vi "MC5e Calculate_Squad.vi"(6 "index":i32, 7 "Mode":T1, 11 "Input Squad":T3={"Squad Name"="", "# Soldiers"=1, "Battle Rating"=0, "Flying"=FALSE, "Mounted"=FALSE, "Speed"=3, "Range"=1, "Morale"=0, "Max Endurance"=10, "Current Endurance"=10, "Size"=enum."Medium", "Space Taken"=1, "Difficult Terrain"=[0, 1, 3, 6, 7], "CR"=1, "Special / Notes"=""} {"CR" items=["30", "29", "28", "27", "26", "25", "24", "23", "22", "21", "20", "19", "18", "17", "16", "15", "14", "13", "12", "11", "10", "9", "8", "7", "6", "5", "4", "3", "2", "1", "1/2", "1/4", "1/8"]}) -> (2 "OK Button Disabled?":T2(ring), 3 "output squad":T3={"Squad Name"="", "# Soldiers"=1, "Battle Rating"=0, "Flying"=FALSE, "Mounted"=FALSE, "Speed"=3, "Range"=1, "Morale"=0, "Max Endurance"=10, "Current Endurance"=10, "Size"=enum."Medium", "Space Taken"=1, "Difficult Terrain"=[0, 1, 3, 6, 7], "CR"=1, "Special / Notes"=""} {"CR" items=["30", "29", "28", "27", "26", "25", "24", "23", "22", "21", "20", "19", "18", "17", "16", "15", "14", "13", "12", "11", "10", "9", "8", "7", "6", "5", "4", "3", "2", "1", "1/2", "1/4", "1/8"]})   [LabVIEW 2020]
uses:
  MC5e Squad_Info.ctl
  MC5e Size_Categories.ctl
  MC53 Editor modes.ctl
panel:
  # "Squads are restricted to one type of soldier (i.e  Archers) and all of the same level.\nIf you want mixed CR or mixed types, use multiple squads."
  # "Squads are restricted to one type of soldier (i.e  Archers) and all of the same level.\nIf you want mixed CR or mixed types, use multiple squads."
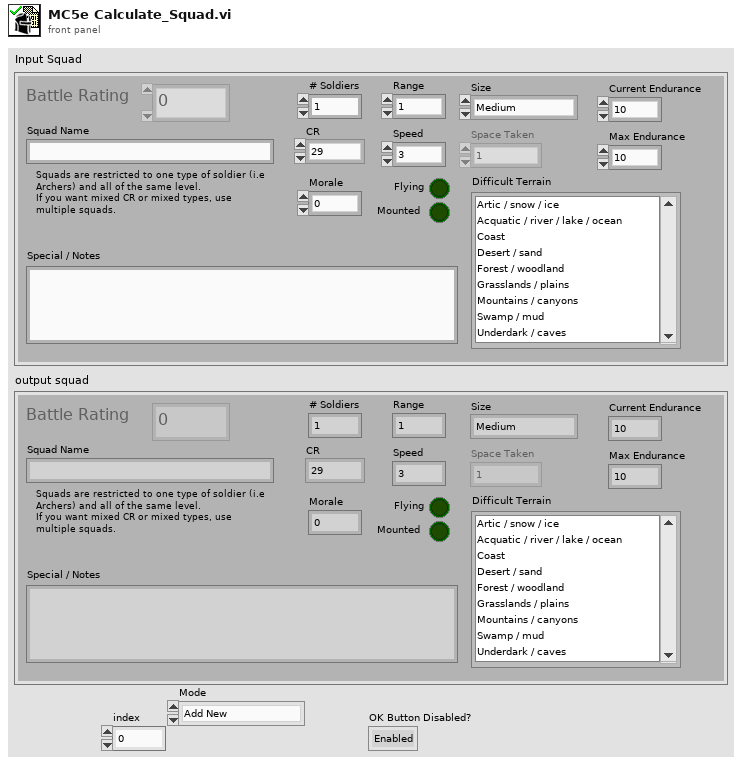
[diagram p1: front panel]
types:
  T1 = typedef "MC53 Editor modes.ctl" = enum16{"Add New", "Copy Selected", "Delete Selected", "Edit Selected"}
  T2 = enum8{"Enabled", "Disabled", "Disabled and Grayed Out"}
  T3 = typedef "MC5e Squad_Info.ctl" = cluster{"Squad Name":string, "# Soldiers":u16, "Battle Rating":u16, "Flying":bool, "Mounted":bool, "Speed":u16, "Range":u16, "Morale":i32, "Max Endurance":u16, "Current Endurance":i32, "Size":T4, "Space Taken":u16, "Difficult Terrain":i32[], "CR":u16, "Special / Notes":string}
  T4 = typedef "MC5e Size_Categories.ctl" = enum16{"Tiny", "Small", "Medium", "Large", "Huge", "Gargantuan"}
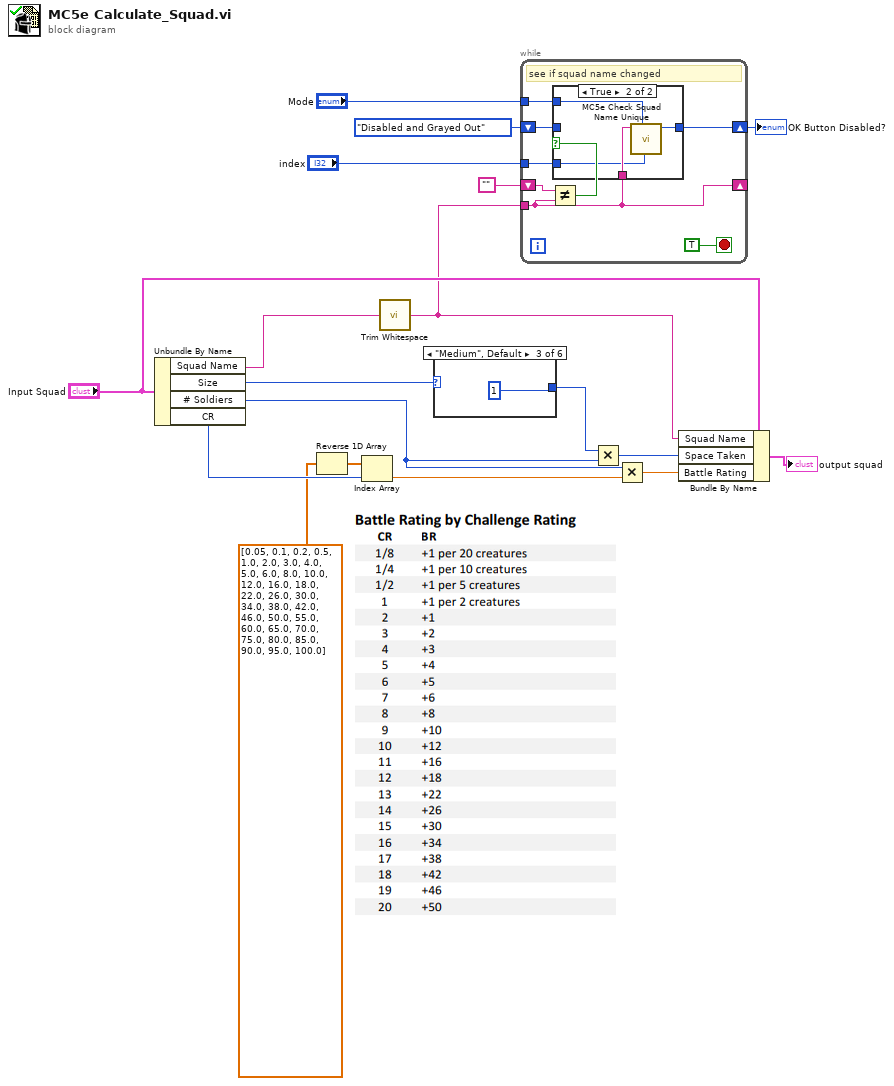
[diagram p0: block diagram]
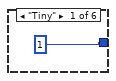
[diagram p3: hidden frame]
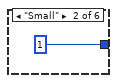
[diagram p4: hidden frame]
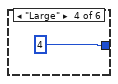
[diagram p5: hidden frame]
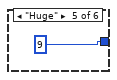
[diagram p6: hidden frame]
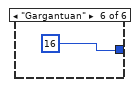
[diagram p7: hidden frame]
diagram:
  n1 = Unbundle By Name("Input Squad") -> ("Squad Name"=w9:string, "Size"=w17:T4, "# Soldiers"=w13:u16, "CR"=w11:u16)
  n2 = Reverse 1D Array(array=dbl[] [0.05, 0.1, 0.2, 0.5, 1.0, 2.0, 3.0, 4.0, 5.0, 6.0, 8.0, 10.0, 12.0, 16.0, 18.0, 22.0, 26.0, 30.0, 34.0, 38.0, 42.0, 46.0, 50.0, 55.0, 60.0, 65.0, 70.0, 75.0, 80.0, 85.0, 90.0, 95.0, 100.0]) -> (reversed array=w3:dbl[])
  n3 = Index Array(array=w3, index=w11) -> (element=w10:dbl)
  n4 = call <vilib>:"Trim Whitespace.vi"("string"=w9) -> ("trimmed string"=w7:string)  [unwired: 1 in]
  n5 = case shown="\"Medium\", Default" w17 {
    tunnel: [1 1 1 4 9 16] -> w16
    frame "Tiny" {
    }
    frame "Small" {
    }
    frame "Medium", Default {
    }
    frame "Large" {
    }
    frame "Huge" {
    }
    frame "Gargantuan" {
    }
  }
  n6 = while {
    shift-right: [w29] -> _
    shift-left: "" -> [w31]
    tunnel: w7 -> [w29]
    shift-right: [w28] -> w6
    shift-left: T2."Disabled and Grayed Out" ("OK Button Disabled?") -> [w27]
    tunnel: "index" -> [w26]
    tunnel: "Mode" -> [w25]
    stop <- TRUE stop-if-true
    # "see if squad name changed"
    n7 = Not Equal?(x=w31, y=w29) -> (x != y?=w30:bool)
    n8 = case shown="True" w30 {
      tunnel: w29 -> [_ w37]
      tunnel: [w33 w36] -> w28
      tunnel: w27 -> [w33 _]
      tunnel: w26 -> [_ w35]
      tunnel: w25 -> [_ w34]
      frame False {
      }
      frame True {
        n9 = call "MC5e Check Squad Name Unique.vi"("index"=w35, "Mode"=w34, "Squad Name"=w37) -> ("OK Button Disabled?"=w36:T2)  [unwired: 7 in, 1 out]
      }
    }
  }
  "OK Button Disabled?" <- w6
  n10 = Multiply(x=w16, y=w13) -> (x*y=w15:i32)
  n11 = Multiply(x=w13, y=w10) -> (x*y=w12:dbl)
  n12 = Bundle By Name(cluster="Input Squad", "Squad Name"=w7, "Space Taken"=w15, "Battle Rating"=w12) -> (→"output squad":T3)
